vi "JHOC Data Processor.vi"(5 "Statemachine Data IN":T7={"Impulse Positions"=[], "No. Imp"=0, "Parameter Time Series"=[], "Parameter Impuls Series"=[], "Experiment Parameters"={"Freq"=0.0, "Vel"=0, "Acc"=0, "Stimulus"=""}, "Autosort File"=refnum, "Data File"={"Data Channels"=[], "Sample Rate"=0, "Channel List"=[]}, "Experiment data path"=path "/Macintosh HD/Users/patrick/Studium/Diploma Thesis/Data Analysis", "Image data path"=path "/Macintosh HD/Users/patrick/Studium/Diploma Thesis/Data Analysis", "LVS data path"=path "/Macintosh HD/Users/patrick/Studium/Diploma Thesis/Data Analysis", "Raw copy path"=path "/Macintosh HD/Users/patrick/Studium/Diploma Thesis/Data Analysis", "filename"="No file selected", "desaccading parameters"={"Tolerance"=0, "Acc Range"=0.0, "Sample Rate"=0, "Impulse Plane 2"=enum."Other", "Impulse dir"=FALSE}, "Experiment Parameters 2"={"Subject"="", "Strain"="", "Rotation plane"="", "Experimenter"="", "Trial"=0.0, "Time"=0.0}, "Excel"={"Excel._Application"=refnum, "Use Excel"=FALSE, "Worksheet SINE"=refnum, "Row SINE"=0, "Worksheet TRANS"=refnum, "Row TRANS"=0}, "Session Config File"=refnum, "Autosort Parameter Set"=1, "EMA Version"="", "desacc "={"Threshold 1 [Acc]"=1617.080808080808, "Threshold 2 [% of TH1]"=67, "tolerance"=5, "Search WD "=0.19090909090909092, " always use TH2"=TRUE, "Range"=3.2323232323232323, "Max time"=200.0, "Min time"=20.0, "Velocity Threshold"=67}, "Cycle Nr for Saccades"={"POS"=0, "NEG"=0}, "calibration name"="No file selected"} {"Parameter Time Series"."time offset" format="%.3f"; "Parameter Time Series"."Gain" format="%.1f"; "Parameter Time Series"."Offset" format="%.1f"; "Parameter Time Series"."List 1" items=["Motor-Pos", "Motor-Vel", "Lx Position-in-Head", "Ly Position-in-Head", "Lz Position-in-Head", "Lx Velocity-in-Head", "Ly Velocity-in-Head", "Lz Velocity-in-Head", "Ll Velocity-in-Head", "Lr Velocity-in-Head", "Lx Accel-in-Head", "Ly Accel-in-Head", "Lz Accel-in-Head", "Rx Position-in-Head", "Ry Position-in-Head", "Rz Position-in-Head", "Rx Velocity-in-Head", "Ry Velocity-in-Head", "Rz Velocity-in-Head", "Rl Velocity-in-Head", "Rr Velocity-in-Head", "Rx Accel-in-Head", "Ry Accel-in-Head", "Rz Accel-in-Head", "Global Trigger", "", "", ""]; "Parameter Impuls Series"."Gain" format="%.1f"; "Parameter Impuls Series"."Offset" format="%.1f"}, 8 "DC-File":path) -> (4 "Statemachine Data IN 2":T7={"Impulse Positions"=[], "No. Imp"=0, "Parameter Time Series"=[], "Parameter Impuls Series"=[], "Experiment Parameters"={"Freq"=0.0, "Vel"=0, "Acc"=0, "Stimulus"=""}, "Autosort File"=refnum, "Data File"={"Data Channels"=[], "Sample Rate"=0, "Channel List"=[]}, "Experiment data path"=path "/Macintosh HD/Users/patrick/Studium/Diploma Thesis/Data Analysis", "Image data path"=path "/Macintosh HD/Users/patrick/Studium/Diploma Thesis/Data Analysis", "LVS data path"=path "/Macintosh HD/Users/patrick/Studium/Diploma Thesis/Data Analysis", "Raw copy path"=path "/Macintosh HD/Users/patrick/Studium/Diploma Thesis/Data Analysis", "filename"="No file selected", "desaccading parameters"={"Tolerance"=0, "Acc Range"=0.0, "Sample Rate"=0, "Impulse Plane 2"=enum."Other", "Impulse dir"=FALSE}, "Experiment Parameters 2"={"Subject"="", "Strain"="", "Rotation plane"="", "Experimenter"="", "Trial"=0.0, "Time"=0.0}, "Excel"={"Excel._Application"=refnum, "Use Excel"=FALSE, "Worksheet SINE"=refnum, "Row SINE"=0, "Worksheet TRANS"=refnum, "Row TRANS"=0}, "Session Config File"=refnum, "Autosort Parameter Set"=1, "EMA Version"="", "desacc "={"Threshold 1 [Acc]"=7000.0, "Threshold 2 [% of TH1]"=60, "tolerance"=3, "Search WD "=0.1, " always use TH2"=FALSE, "Range"=2.0, "Max time"=120.0, "Min time"=20.0, "Velocity Threshold"=150}, "Cycle Nr for Saccades"={"POS"=0, "NEG"=0}, "calibration name"="No file selected"} {"Parameter Time Series"."time offset" format="%.3f"; "Parameter Time Series"."Gain" format="%.1f"; "Parameter Time Series"."Offset" format="%.1f"; "Parameter Time Series"."List 1" items=["Motor-Pos", "Motor-Vel", "Lx Position-in-Head", "Ly Position-in-Head", "Lz Position-in-Head", "Lx Velocity-in-Head", "Ly Velocity-in-Head", "Lz Velocity-in-Head", "Ll Velocity-in-Head", "Lr Velocity-in-Head", "Lx Accel-in-Head", "Ly Accel-in-Head", "Lz Accel-in-Head", "Rx Position-in-Head", "Ry Position-in-Head", "Rz Position-in-Head", "Rx Velocity-in-Head", "Ry Velocity-in-Head", "Rz Velocity-in-Head", "Rl Velocity-in-Head", "Rr Velocity-in-Head", "Rx Accel-in-Head", "Ry Accel-in-Head", "Rz Accel-in-Head", "Global Trigger", "", "", ""]; "Parameter Impuls Series"."Gain" format="%.1f"; "Parameter Impuls Series"."Offset" format="%.1f"})   [LabVIEW 2016]
uses:
  core/type-defs/TD_Statemachine-Data.ctl
  core/type-defs/TD_Time Series.ctl
  core/type-defs/TD_Impulse Parameter.ctl
  JHOC state.ctl
  core/core.lvlib
panel:
  in  "Tab Control":T1(tab)
  in  "Selected Calibration File":string
  in  "Calibration File":bool
  out "Processing":bool
  in  "3D Convention":T2(ring)=enum."Rotation Vectors"
  in  "Selected Data File":string
  in  "Data File 2":bool
  in  "Start Processing":bool
  in  "Calibration Channels":u16[][](array[ring])=[[16, 13, 10, 7, 4, 1], [15, 12, 9, 6, 3, 0], [17, 14, 11, 8, 5, 2]] items=["coil_HDX", "coil_HDY", "coil_HDZ", "coil_HTX", "coil_HTY", "coil_HTZ", "coil_LDX", "coil_LDY", "coil_LDZ", "coil_LTX", "coil_LTY", "coil_LTZ", "coil_RDX", "coil_RDY", "coil_RDZ", "coil_RTX", "coil_RTY", "coil_RTZ", "Target Hor", "Target Ver", "Target on/off", "aux input 1", "aux input 2"]
  in  "Cosines fixed":i16[][](array[numeric])
  in  "Sub Sample Once":bool
  in  "Manually enter the Field Gains":bool
  in  "Parameter Time Series":T3 {"time offset" format="%.3f"; "Gain" format="%.1f"; "Offset" format="%.1f"; "List 1" items=["Hz Position-in-Head", "Hz Velocity-in-Head", "Hy Position-in-Head", "Hy Velocity-in-Head", "Hx Position-in-Head", "Hx Velocity-in-Head", "Hl Velocity-in-Head", "Hr Velocity-in-Head", "Lx Position-in-Head", "Ly Position-in-Head", "Lz Position-in-Head", "Lx Velocity-in-Head", "Ly Velocity-in-Head", "Lz Velocity-in-Head", "Ll Velocity-in-Head", "Lr Velocity-in-Head", "Rx Position-in-Head", "Ry Position-in-Head", "Rz Position-in-Head", "Rx Velocity-in-Head", "Ry Velocity-in-Head", "Rz Velocity-in-Head", "Rl Velocity-in-Head", "Rr Velocity-in-Head", "Target on/off", "aux input 1", "aux input 2", " ", "", "", "", "Target Hor", "Target Ver", ""]}
  in  "Parameter Impuls Series":T4=[{"Color"=4652800, "Visible"=TRUE, "Channel"=1, "Invert"=FALSE, "Desaccade"=FALSE, "Offset"=0.0, "Gain"=1.0}, {"Color"=16860, "Visible"=TRUE, "Channel"=13, "Invert"=TRUE, "Desaccade"=FALSE, "Offset"=0.0, "Gain"=1.0}, {"Color"=16711680, "Visible"=TRUE, "Channel"=21, "Invert"=TRUE, "Desaccade"=FALSE, "Offset"=0.0, "Gain"=1.0}] {"Gain" format="%.1f"; "Offset" format="%.1f"; "Channel" items=["Hz Position-in-Head", "Hz Velocity-in-Head", "Hy Position-in-Head", "Hy Velocity-in-Head", "Hx Position-in-Head", "Hx Velocity-in-Head", "Hl Velocity-in-Head", "Hr Velocity-in-Head", "Lx Position-in-Head", "Ly Position-in-Head", "Lz Position-in-Head", "Lx Velocity-in-Head", "Ly Velocity-in-Head", "Lz Velocity-in-Head", "Ll Velocity-in-Head", "Lr Velocity-in-Head", "Rx Position-in-Head", "Ry Position-in-Head", "Rz Position-in-Head", "Rx Velocity-in-Head", "Ry Velocity-in-Head", "Rz Velocity-in-Head", "Rl Velocity-in-Head", "Rr Velocity-in-Head", "Target on/off", "aux input 1", "aux input 2", " ", "", "", "", "Target Hor", "Target Ver", ""]}
  in  "Export Channel List":u16[](array[ring])=[2, 11, 1, 10, 0, 9, 12, 13, 3, 4, 5, 14, 15, 16, 17, 18, 6, 7, 8, 19, 20, 21, 22, 23, 26, 27, 28, 29, 30, 31, 34, 24, 25, 38] items=["Hx Position-in-Head", "Hy Position-in-Head", "Hz Position-in-Head", "Lx Position-in-Head", "Ly Position-in-Head", "Lz Position-in-Head", "Rx Position-in-Head", "Ry Position-in-Head", "Rz Position-in-Head", "Hx Velocity-in-Head", "Hy Velocity-in-Head", "Hz Velocity-in-Head", "Hl Velocity-in-Head", "Hr Velocity-in-Head", "Lx Velocity-in-Head", "Ly Velocity-in-Head", "Lz Velocity-in-Head", "Ll Velocity-in-Head", "Lr Velocity-in-Head", "Rx Velocity-in-Head", "Ry Velocity-in-Head", "Rz Velocity-in-Head", "Rl Velocity-in-Head", "Rr Velocity-in-Head", "Target Hor", "Target Ver", "Target on/off", "aux input 1", "aux input 2", " "]
  in  "Additional channels":T5(array[cluster])=[{"offset"=0.0, "scale"=1.0, "channel select"=18}, {"offset"=0.0, "scale"=1.0, "channel select"=19}, {"offset"=0.0, "scale"=0.0060606, "channel select"=20}, {"offset"=0.0, "scale"=1.0, "channel select"=21}, {"offset"=0.0, "scale"=1.0, "channel select"=22}] {"channel select" items=["coil_HDX", "coil_HDY", "coil_HDZ", "coil_HTX", "coil_HTY", "coil_HTZ", "coil_LDX", "coil_LDY", "coil_LDZ", "coil_LTX", "coil_LTY", "coil_LTZ", "coil_RDX", "coil_RDY", "coil_RDZ", "coil_RTX", "coil_RTY", "coil_RTZ", "Target Hor", "Target Ver", "Target on/off", "aux input 1", "aux input 2"]; "scale" format="%.7f"; "offset" format="%.2f"}
  in  "Coil Channels":u16[][](array[ring])=[[0, 6, 12], [1, 7, 13], [2, 8, 14], [3, 9, 15], [4, 10, 16], [5, 11, 17]] items=["coil_HDX", "coil_HDY", "coil_HDZ", "coil_HTX", "coil_HTY", "coil_HTZ", "coil_LDX", "coil_LDY", "coil_LDZ", "coil_LTX", "coil_LTY", "coil_LTZ", "coil_RDX", "coil_RDY", "coil_RDZ", "coil_RTX", "coil_RTY", "coil_RTZ", "Target Hor", "Target Ver", "Target on/off", "aux input 1", "aux input 2"]
  in  "DAQ data setup":T6={"Input Channels"=[{"channel name"="coil_HDX", "channel number"=0.0}, {"channel name"="coil_HDY", "channel number"=1.0}, {"channel name"="coil_HDZ", "channel number"=2.0}, {"channel name"="coil_HTX", "channel number"=3.0}, {"channel name"="coil_HTY", "channel number"=4.0}, {"channel name"="coil_HTZ", "channel number"=5.0}, {"channel name"="coilLDX", "channel number"=6.0}, {"channel name"="coil_LDY", "channel number"=7.0}, {"channel name"="coil_LDZ", "channel number"=8.0}, {"channel name"="coil_LTX", "channel number"=9.0}, {"channel name"="coil_LTY", "channel number"=10.0}, {"channel name"="coil_LTZ", "channel number"=11.0}, {"channel name"="coil_RDX", "channel number"=12.0}, {"channel name"="coil_RDY", "channel number"=13.0}, {"channel name"="coil_RDZ", "channel number"=14.0}, {"channel name"="coil_RTX", "channel number"=15.0}, {"channel name"="coil_RTY", "channel number"=16.0}, {"channel name"="coil_RTZ", "channel number"=17.0}], "Sample Rate"=1000.0}
  in  "plot length":i32=15000
  in  "Channel \nplot":u16[](array[ring])=[7, 8, 10, 11, 1, 2] items=["coil_HDX", "coil_HDY", "coil_HDZ", "coil_HTX", "coil_HTY", "coil_HTZ", "coil_LDX", "coil_LDY", "coil_LDZ", "coil_LTX", "coil_LTY", "coil_LTZ", "coil_RDX", "coil_RDY", "coil_RDZ", "coil_RTX", "coil_RTY", "coil_RTZ", "Target Hor", "Target Ver", "Target on/off", "aux input 1", "aux input 2"]
  out "DAQ calibration setup":T6={"Input Channels"=[{"channel name"="chairpos", "channel number"=1.0}, {"channel name"="coil_RDY", "channel number"=2.0}, {"channel name"="coil_RDZ", "channel number"=3.0}, {"channel name"="coil_RDX", "channel number"=4.0}, {"channel name"="coil_RTY", "channel number"=5.0}, {"channel name"="coil_RTZ", "channel number"=6.0}, {"channel name"="coil_RTX", "channel number"=7.0}, {"channel name"="coil_HDY", "channel number"=8.0}, {"channel name"="coil_HDZ", "channel number"=9.0}, {"channel name"="coil_HDX", "channel number"=10.0}, {"channel name"="coil_LDY", "channel number"=11.0}, {"channel name"="coil_LDZ", "channel number"=12.0}, {"channel name"="coil_LDX", "channel number"=13.0}, {"channel name"="coil_LTY", "channel number"=14.0}, {"channel name"="coil_LTZ", "channel number"=15.0}, {"channel name"="coil_LTX", "channel number"=16.0}, {"channel name"="coil_HTY", "channel number"=17.0}, {"channel name"="coil_HTZ", "channel number"=18.0}, {"channel name"="coil_HTX", "channel number"=19.0}, {"channel name"="chairvel", "channel number"=20.0}, {"channel name"="button", "channel number"=22.0}, {"channel name"="accel_head", "channel number"=25.0}, {"channel name"="ascension_x", "channel number"=33.0}, {"channel name"="ascension_y", "channel number"=34.0}, {"channel name"="ascension_z", "channel number"=35.0}, {"channel name"="ascension_q0", "channel number"=36.0}, {"channel name"="ascension_q1", "channel number"=37.0}, {"channel name"="ascension_q2", "channel number"=38.0}, {"channel name"="ascension_q3", "channel number"=39.0}, {"channel name"="led_code", "channel number"=40.0}], "Sample Rate"=1000.0}
  in  "Data File":T8 {"Data -> Plot" format="%.2f"; "Data -> Additional" format="%.2f"; "Data -> 3D Coil" format="%.2f"}
  in  "All Data":T9={"Data Channels"=[], "Sample Rate"=0, "Channel List"=["Hx Position-in-Head", "Hy Position-in-Head", "Hz Position-in-Head", "Lx Position-in-Head", "Ly Position-in-Head", "Lz Position-in-Head", "Rx Position-in-Head", "Ry Position-in-Head", "Rz Position-in-Head", "Hx Velocity-in-Head", "Hy Velocity-in-Head", "Hz Velocity-in-Head", "Hl Velocity-in-Head", "Hr Velocity-in-Head", "Lx Velocity-in-Head", "Ly Velocity-in-Head", "Lz Velocity-in-Head", "Ll Velocity-in-Head", "Lr Velocity-in-Head", "Rx Velocity-in-Head", "Ry Velocity-in-Head", "Rz Velocity-in-Head", "Rl Velocity-in-Head", "Rr Velocity-in-Head", "coil_HTX", "chairvel", "button", " "]} {"Data Channels" format="%.2f"}
  # "NOTE: EMPTY STRING ALWAYS AT END"
  # "JHOC Data Processor"
  # "By Americo A. Migliaccio\nand Patrick P. Huebner \nMarch 2014 ver 2.0"
  # "Head coil                             Left eye coil                        Right eye coil"
  # "DX\n\nDY\n\nDZ\n\nTX\n\nTY\n\nTZ"
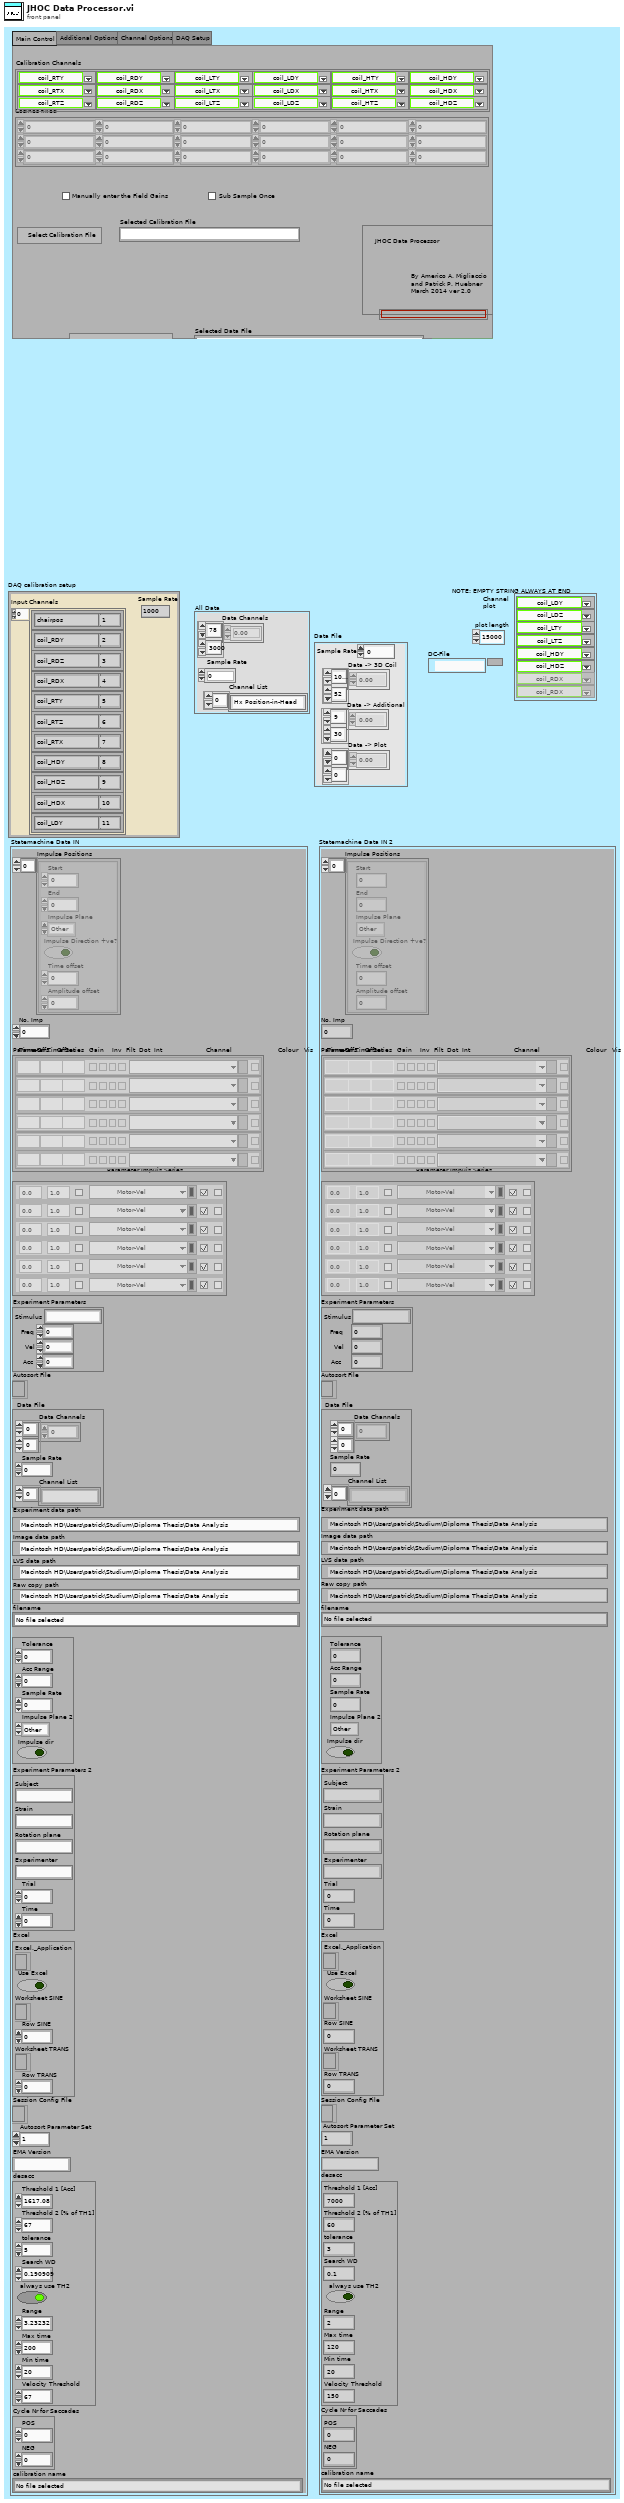
[diagram p1: front panel]
types:
  T1 = enum32{"Main Control", "Additional Options", "Channel Options", "DAQ Setup"}
  T2 = enum16{"Rotation Matrix", "Rotation Vectors", "Quaternions", "Fick Angles", "Helmholtz Angles"}
  T3 = typedef "core.lvlib/TD_Time Series.ctl" = cluster{"time offset":dbl, "Offset":dbl, "Gain":dbl, "inverse":bool, "filter data":bool, "dots":bool, "interpolate":bool, "List 1":u16, "Color Box":u32, "Boolean":bool}[]
  T4 = typedef "core.lvlib/TD_Impulse Parameter.ctl" = cluster{"Color":u32, "Visible":bool, "Channel":u16, "Invert":bool, "Desaccade":bool, "Offset":dbl, "Gain":dbl}[]
  T5 = cluster{"offset":dbl, "scale":dbl, "channel select":u16}[]
  T6 = cluster{"Input Channels":cluster{"channel name":string, "channel number":dbl}[], "Sample Rate":dbl}
  T7 = typedef "core.lvlib/TD_Statemachine-Data.ctl" = cluster{"Impulse Positions":cluster{"Start":i32, "End":i32, "Impulse Plane":enum16{"Other", "Yaw", "Pitch", "Roll", "LARP", "RALP"}, "Impulse Direction +ve?":bool, "Time offset":i32, "Amplitude offset":dbl}[], "No. Imp":i32, "Parameter Time Series":T3, "Parameter Impuls Series":T4, "Experiment Parameters":cluster{"Freq":dbl, "Vel":i32, "Acc":i32, "Stimulus":string}, "Autosort File":refnum<file>, "Data File":cluster{"Data Channels":dbl[][], "Sample Rate":i32, "Channel List":string[]}, "Experiment data path":path, "Image data path":path, "LVS data path":path, "Raw copy path":path, "filename":string, "desaccading parameters":cluster{"Tolerance":i32, "Acc Range":dbl, "Sample Rate":i32, "Impulse Plane 2":enum16{"Other", "Yaw", "Pitch", "Roll", "LARP", "RALP"}, "Impulse dir":bool}, "Experiment Parameters 2":cluster{"Subject":string, "Strain":string, "Rotation plane":string, "Experimenter":string, "Trial":dbl, "Time":dbl}, "Excel":cluster{"Excel._Application":refnum<k7>, "Use Excel":bool, "Worksheet SINE":refnum<k7>, "Row SINE":i32, "Worksheet TRANS":refnum<k7>, "Row TRANS":i32}, "Session Config File":refnum<file>, "Autosort Parameter Set":i32, "EMA Version":string, "desacc ":cluster{"Threshold 1 [Acc]":dbl, "Threshold 2 [% of TH1]":i32, "tolerance":i32, "Search WD ":dbl, " always use TH2":bool, "Range":dbl, "Max time":dbl, "Min time":dbl, "Velocity Threshold":i32}, "Cycle Nr for Saccades":cluster{"POS":i32, "NEG":i32}, "calibration name":string}
  T8 = cluster{"Sample Rate":i32, "Data -> 3D Coil":dbl[][], "Data -> Additional":dbl[][], "Data -> Plot":dbl[][]}
  T9 = cluster{"Data Channels":dbl[][], "Sample Rate":i32, "Channel List":string[]}
  T10 = typedef "JHOC state.ctl" = enum16{"Panel Monitoring", "Calculate 6 Field/Int Rot Matrix", "SubSample", "Initialize", "Read 6 Field/Int Calibration File", "Read 6 Field/Int Data File", "Sort 6 Field/Int Channels", "Export Channels", "Stop", "Quit"}
  T11 = enum16{"Position in Space", "Position in Head", "Position in Eye", "Velocity in Space", "Velocity in Head", "Velocity in Eye", "Acceleration in Space", "Acceleration in Head"}
  T12 = cluster{"Freq":dbl, "Vel":i32, "Acc":i32, "Stimulus":string}
  T13 = cluster{"DAQ data setup":cluster{"Input Channels":cluster{"channel name":string, "channel number":dbl}[], "Sample Rate":dbl}, "Coil Channels":u16[][], "Additional channels":cluster{"offset":dbl, "scale":dbl, "channel select":u16}[], "Selected Calibration File":string, "Selected Data File":string, "Cosines fixed":i16[][], "Data File":cluster{"Sample Rate":i32, "Data -> 3D Coil":dbl[][], "Data -> Additional":dbl[][], "Data -> Plot":dbl[][]}, "All Data":cluster{"Data Channels":dbl[][], "Sample Rate":i32, "Channel List":string[]}, "Channel \nplot":u16[], "Calibration Channels":u16[][], "Auto load calibration file":path}
  T14 = cluster{"DAQ calibration setup":cluster{"Input Channels":cluster{"channel name":string, "channel number":dbl}[], "Sample Rate":dbl}, "Calibration Channels":u16[][]}
  T15 = cluster{"channel name":string, "channel number":dbl}[]
  T16 = cluster{"channel name":string, "channel number":dbl}
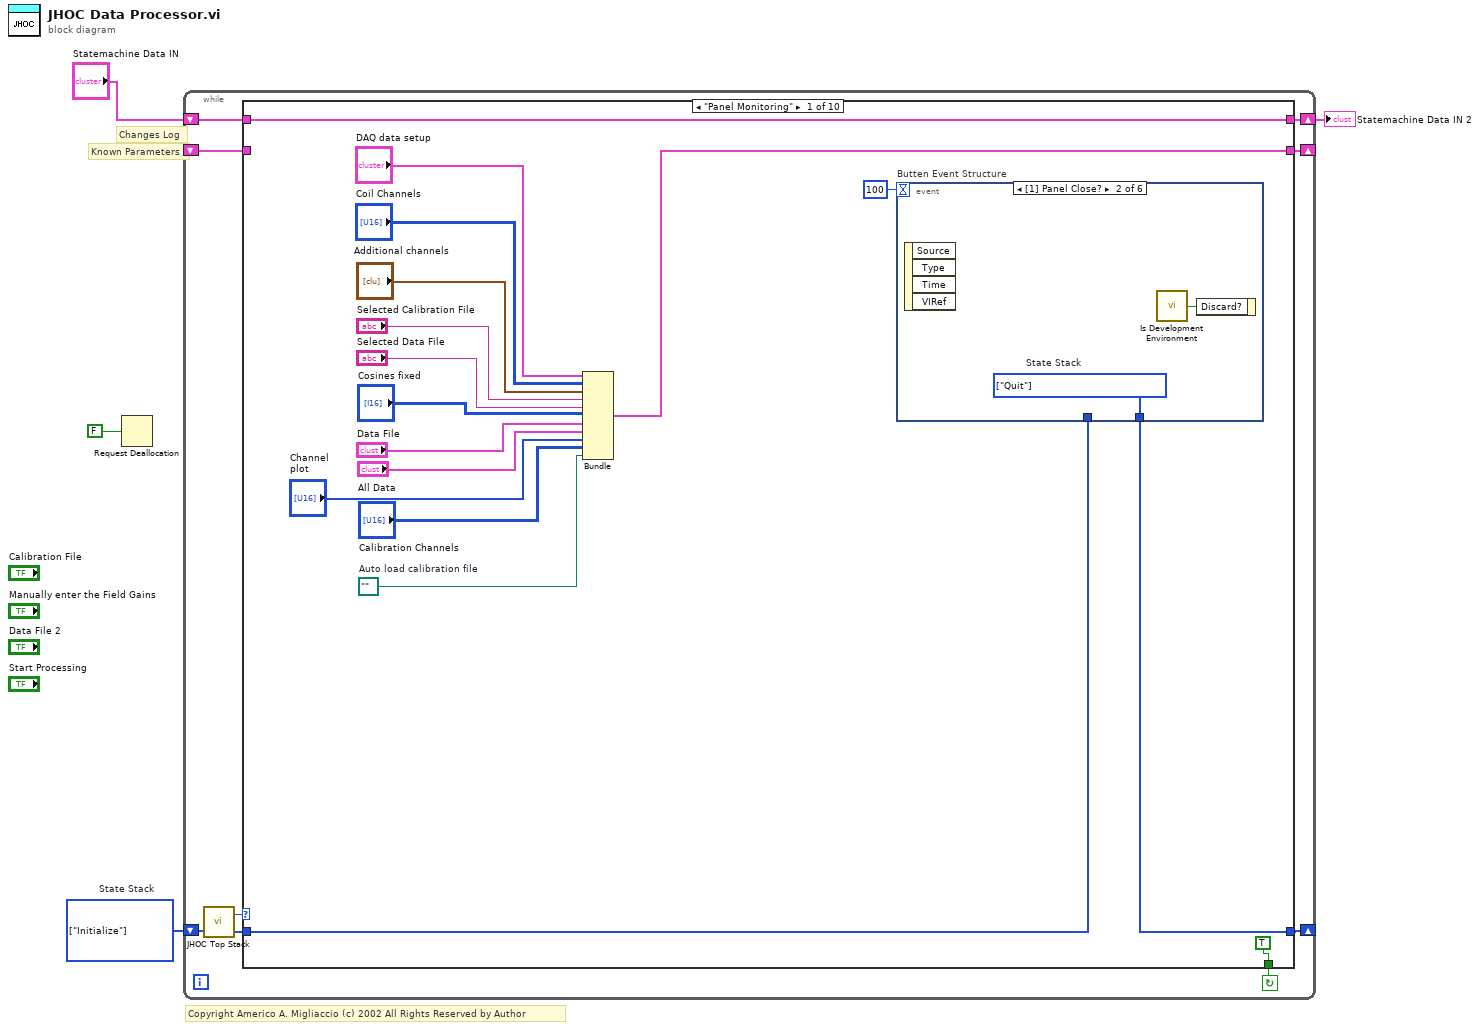
[diagram p0: block diagram]
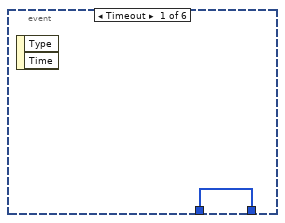
[diagram p2: hidden frame]
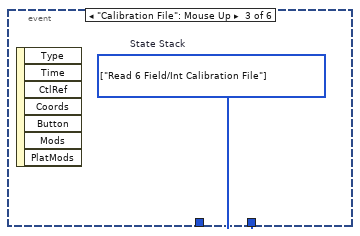
[diagram p3: hidden frame]
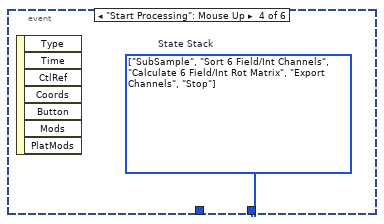
[diagram p4: hidden frame]
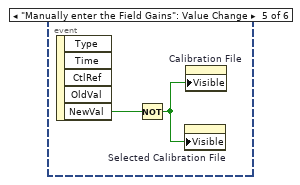
[diagram p5: hidden frame]
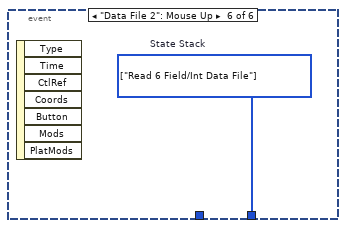
[diagram p6: hidden frame]
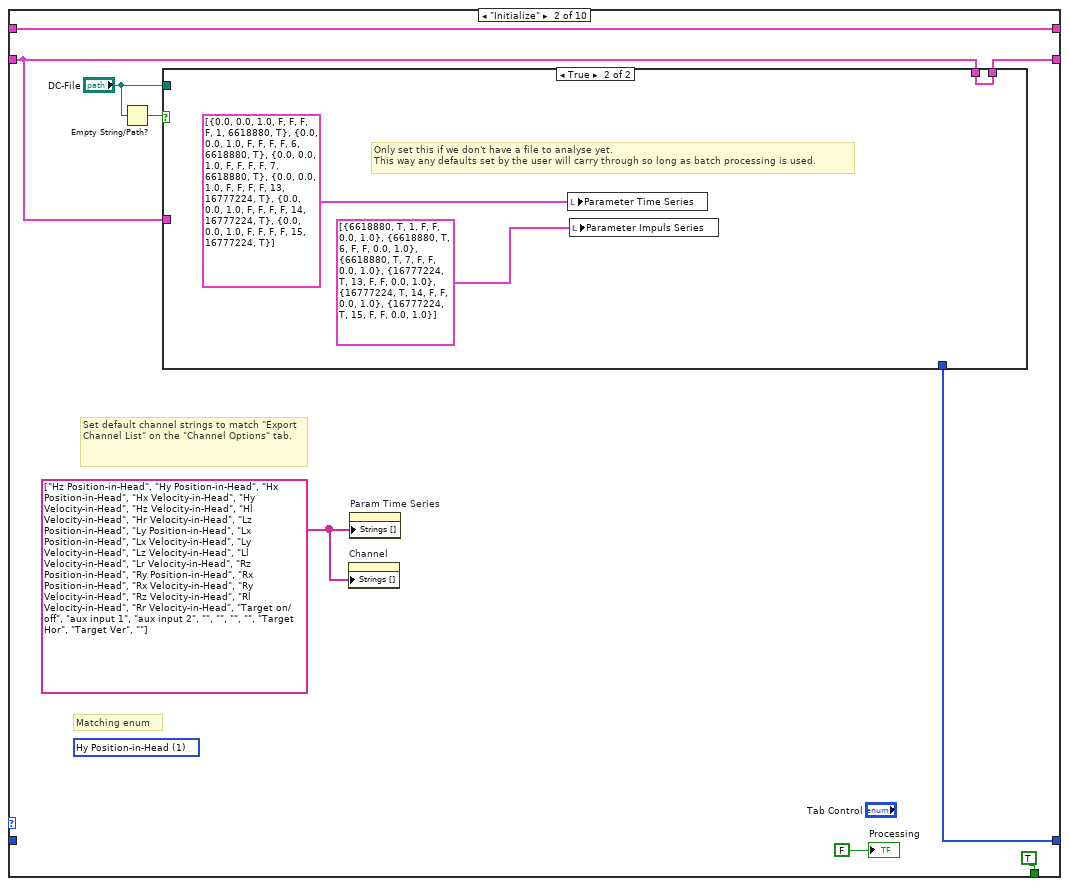
[diagram p7: hidden frame]
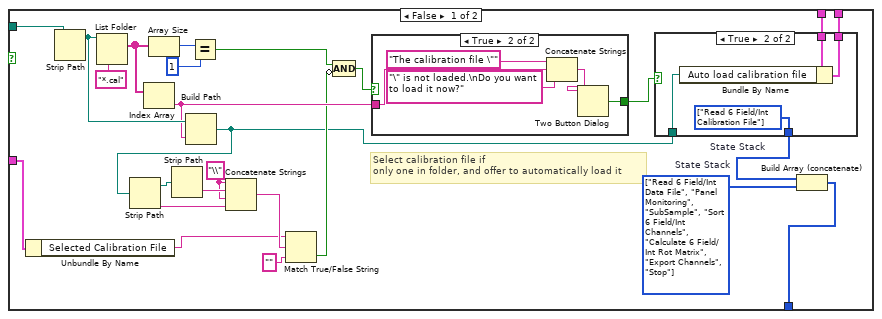
[diagram p8: hidden frame]
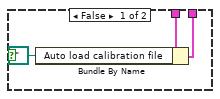
[diagram p9: hidden frame]
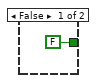
[diagram p10: hidden frame]
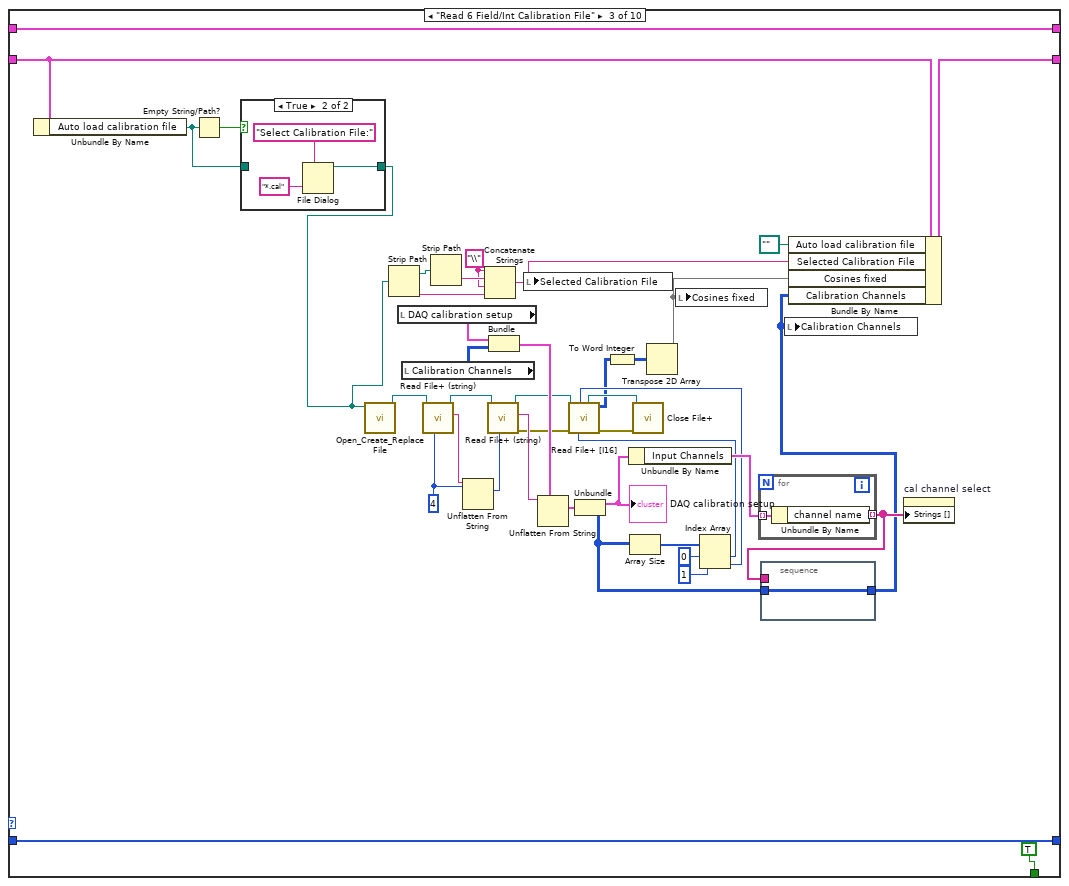
[diagram p11: hidden frame]
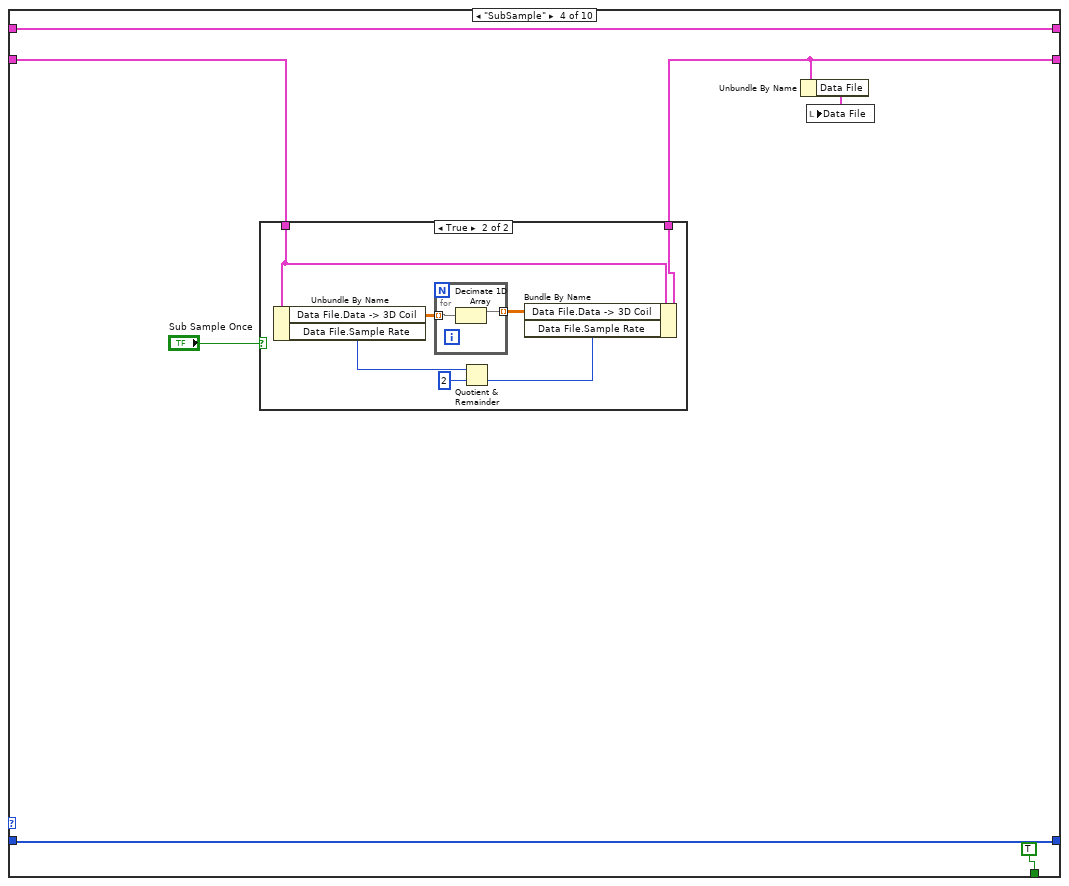
[diagram p13: hidden frame]
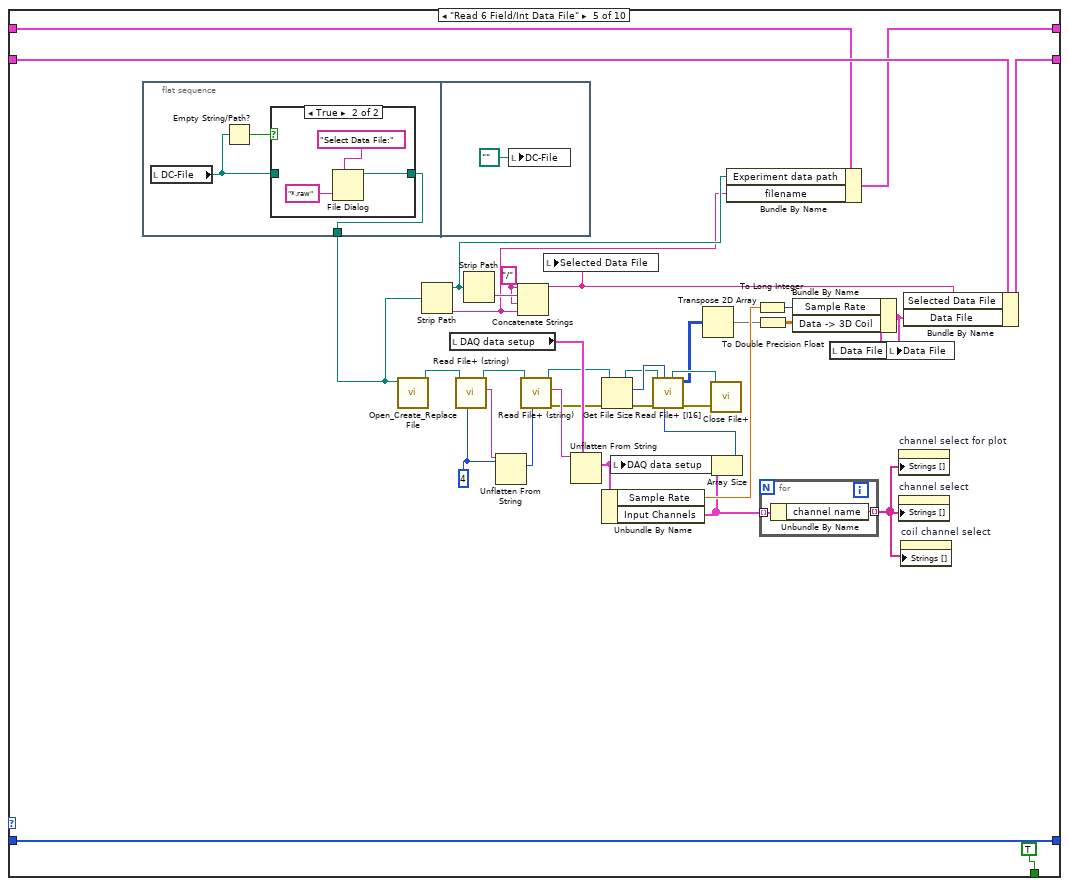
[diagram p15: hidden frame]
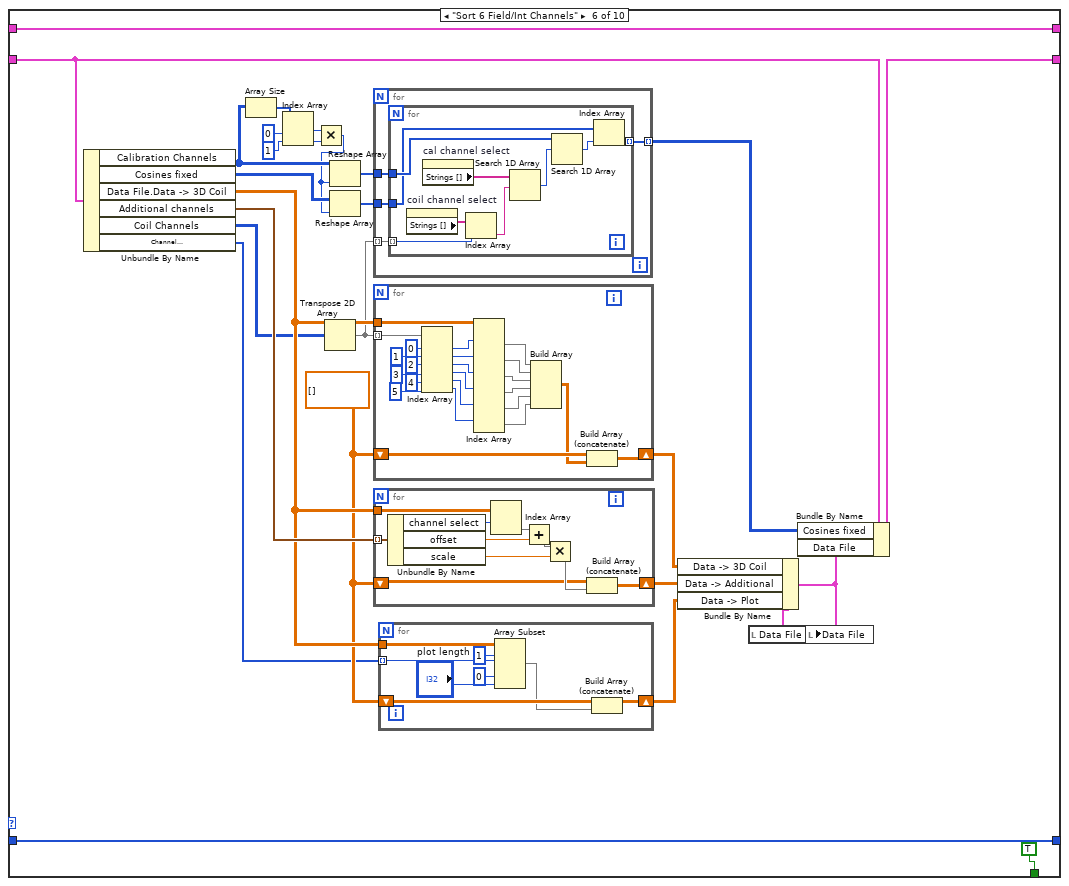
[diagram p17: hidden frame]
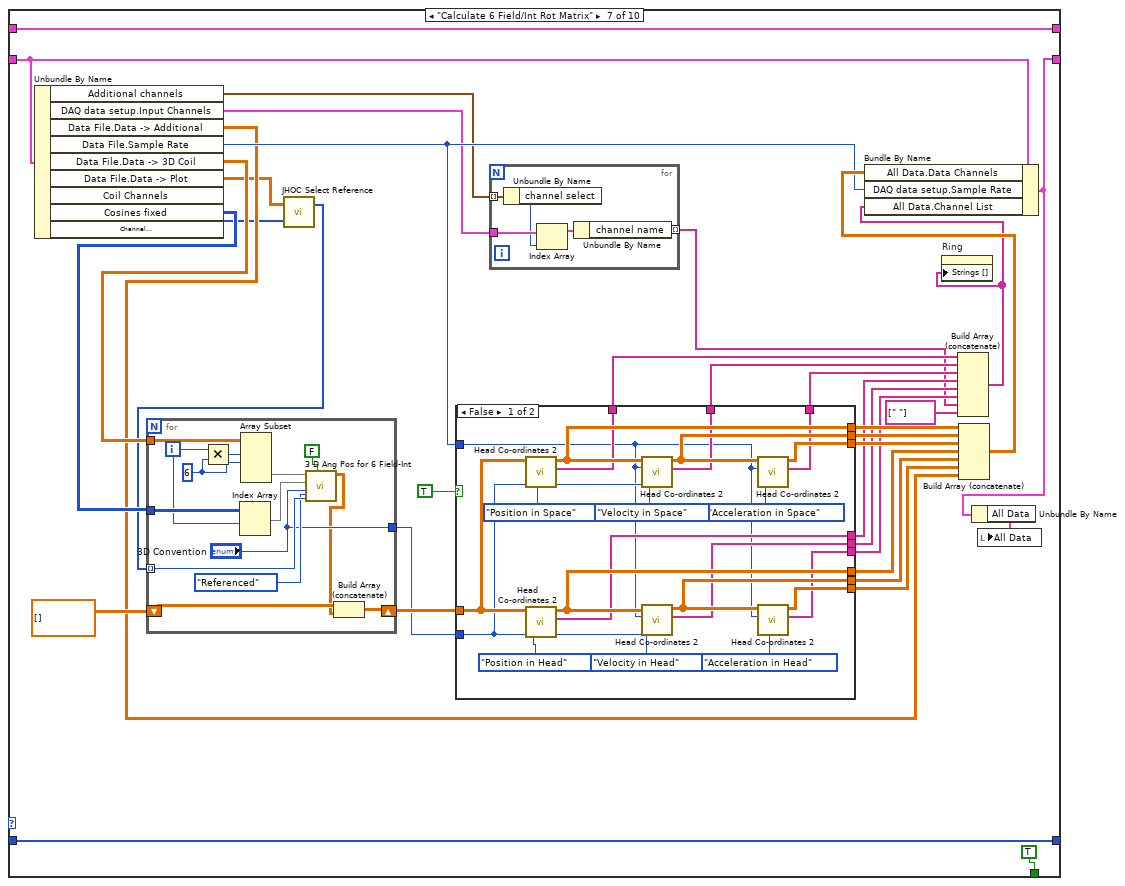
[diagram p18: hidden frame]
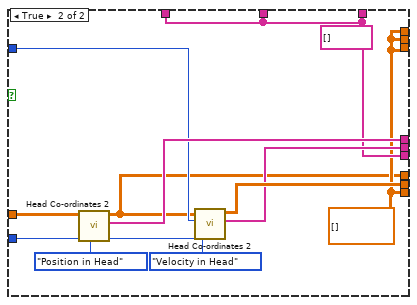
[diagram p19: hidden frame]
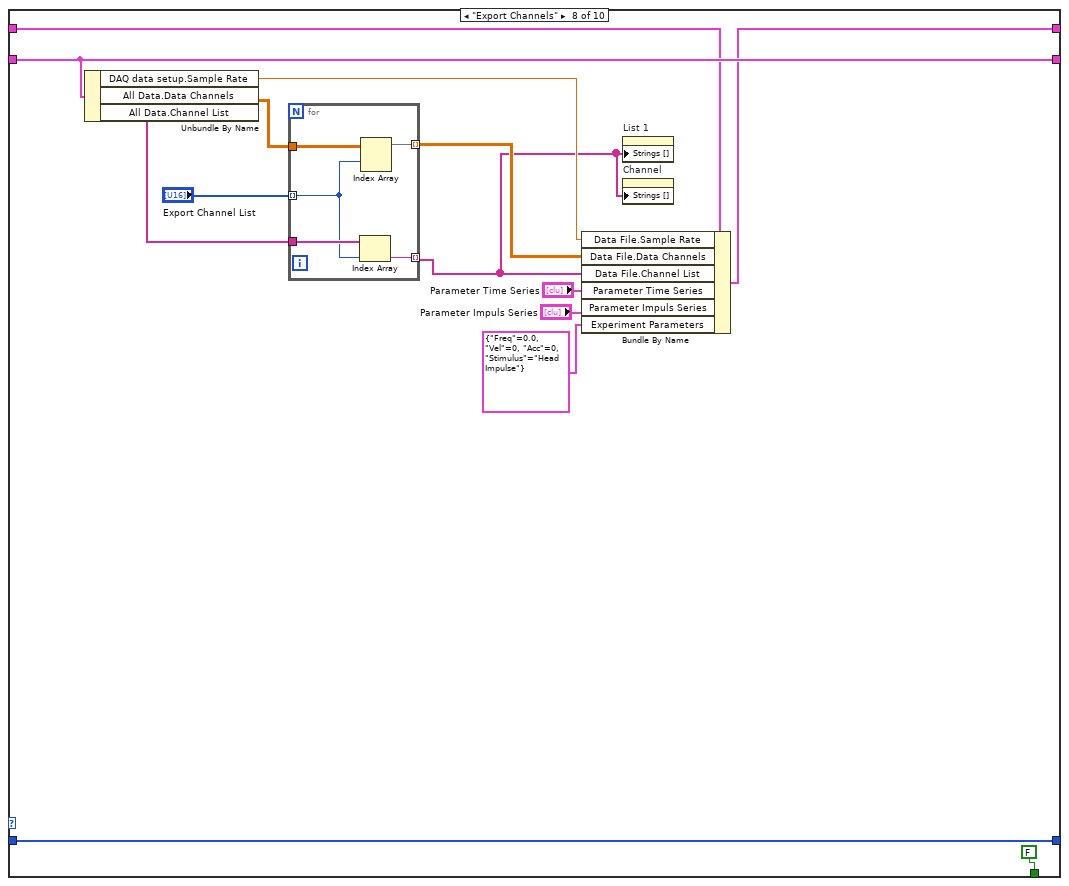
[diagram p20: hidden frame]
diagram:
  w4 = T10[] [enum."Initialize"] items=["Panel Monitoring", "Calculate 6 Field/Int Rot Matrix", "SubSample", "Initialize", "Read 6 Field/Int Calibration File", "Read 6 Field/Int Data File", "Sort 6 Field/Int Channels", "Export Channels", "Stop", "Quit"]  # State Stack
  # "Copyright Americo A. Migliaccio (c) 2002 All Rights Reserved by Author"
  # "Known Parameters"
  # "Changes Log"
  n1 = Request Deallocation(FALSE ("flag")) -> ()
  n2 = while {
    shift-left: _ -> [w9]
    shift-right: [w8] -> _
    shift-left: w4 -> [w13]
    shift-right: [w11] -> _
    shift-right: [w5] -> w1
    shift-left: "Statemachine Data IN" -> [w6]
    stop <- w10 continue-if-true
    n3 = call "JHOC Top Stack.vi"("State Stack (in)"=w13) -> ("State Stack (out)"=w12:T10[], "State 4"=w7:T10)  [unwired: 1 in]
    n4 = case shown="\"Panel Monitoring\"" w7 {
      tunnel: w12 -> [w14 _ w89 w138 w154 w225 w316 w381 w390 w394]
      tunnel: [w17 w41 w89 w138 w154 w225 w316 w381 w390 w394] -> w11
      tunnel: [TRUE TRUE TRUE TRUE TRUE TRUE TRUE FALSE FALSE FALSE] -> w10
      tunnel: [w27 w42 w128 w140 w189 w224 w302 w378 w388 w392] -> w8
      tunnel: w9 -> [_ w40 w94 w142 w188 w226 w312 w378 w388 w392]
      tunnel: w6 -> [w18 w45 w95 w137 w156 w201 w282 w373 w387 w391]
      tunnel: [w18 w45 w95 w137 w155 w201 w282 w372 w387 w391] -> w5
      frame "Panel Monitoring" {
        w15 = path ""  # Auto load calibration file
        n5 = Bundle("DAQ data setup"="DAQ data setup", "Coil Channels"="Coil Channels", "Additional channels"="Additional channels", "Selected Calibration File"="Selected Calibration File", "Selected Data File"="Selected Data File", "Cosines fixed"="Cosines fixed", "Data File"="Data File", "All Data"="All Data", "Channel \nplot"="Channel \nplot", "Calibration Channels"="Calibration Channels", "Auto load calibration file"=w15) -> (w27:T13)  [unwired: 1 in]
        n6 = event "Butten Event Structure" shown="[1] Panel Close?" {
          selector: _ -> [_ _ _ _ _ _]
          dyn-events: _ -> [_ _ _ _ _ _]
          timeout: 100 -> [_ _ _ _ _ _]
          tunnel: [w31 w33 w34 w35 _ w38] -> w17
          tunnel: w14 -> [w31 _ _ _ _ _]
          event Timeout {
            n7 = event-data() -> ()  [unwired: 1 in, 2 out]
          }
          event Panel Close? {
            w33 = T10[] [enum."Quit"] items=["Panel Monitoring", "Calculate 6 Field/Int Rot Matrix", "SubSample", "Initialize", "Read 6 Field/Int Calibration File", "Read 6 Field/Int Data File", "Sort 6 Field/Int Channels", "Export Channels", "Stop", "Quit"]  # State Stack
            n8 = event-data() -> ()  [unwired: 1 in, 4 out]
            n9 = call <userlib>:"Is Development Environment.vi"() -> ("exe?"=w32:bool)  [unwired: 5 in]
            n10 = event-data("Discard?"=w32) -> ()  [unwired: 1 in, 1 out]
          }
          event "Calibration File": Mouse Up {
            w34 = T10[] [enum."Read 6 Field/Int Calibration File"] items=["Panel Monitoring", "Calculate 6 Field/Int Rot Matrix", "SubSample", "Initialize", "Read 6 Field/Int Calibration File", "Read 6 Field/Int Data File", "Sort 6 Field/Int Channels", "Export Channels", "Stop", "Quit"]  # State Stack
            n11 = event-data() -> ()  [unwired: 1 in, 7 out]
          }
          event "Start Processing": Mouse Up {
            w35 = T10[] [enum."SubSample", enum."Sort 6 Field/Int Channels", enum."Calculate 6 Field/Int Rot Matrix", enum."Export Channels", enum."Stop"] items=["Panel Monitoring", "Calculate 6 Field/Int Rot Matrix", "SubSample", "Initialize", "Read 6 Field/Int Calibration File", "Read 6 Field/Int Data File", "Sort 6 Field/Int Channels", "Export Channels", "Stop", "Quit"]  # State Stack
            n12 = event-data() -> ()  [unwired: 1 in, 7 out]
          }
          event "Manually enter the Field Gains": Value Change {
            n13 = event-data() -> ("NewVal"=w36:bool)  [unwired: 1 in, 4 out]
            n14 = Not(x=w36) -> (.not. x?=w37:bool)
            n15 = property on="Selected Calibration File" class="Str"("Visible"=w37) -> ()  [unwired: 2 in, 2 out]
            n16 = property on="Calibration File" class="Bool (strict)"("Visible"=w37) -> ()  [unwired: 2 in, 2 out]
          }
          event "Data File 2": Mouse Up {
            w38 = T10[] [enum."Read 6 Field/Int Data File"] items=["Panel Monitoring", "Calculate 6 Field/Int Rot Matrix", "SubSample", "Initialize", "Read 6 Field/Int Calibration File", "Read 6 Field/Int Data File", "Sort 6 Field/Int Channels", "Export Channels", "Stop", "Quit"]  # State Stack
            n17 = event-data() -> ()  [unwired: 1 in, 7 out]
          }
        }
      }
      frame "Initialize" {
        (unwired) u16 1 items=["Hz Position-in-Head", "Hy Position-in-Head", "Hx Position-in-Head", "Hx Velocity-in-Head", "Hy Velocity-in-Head", "Hz Velocity-in-Head", "Hl Velocity-in-Head", "Hr Velocity-in-Head", "Lx Position-in-Head", "Ly Position-in-Head", "Lz Position-in-Head", "Lx Velocity-in-Head", "Ly Velocity-in-Head", "Lz Velocity-in-Head", "Ll Velocity-in-Head", "Lr Velocity-in-Head", "Rz Position-in-Head", "Ry Position-in-Head", "Rx Position-in-Head", "Rx Velocity-in-Head", "Ry Velocity-in-Head", "Rz Velocity-in-Head", "Rl Velocity-in-Head", "Rr Velocity-in-Head", "Target on/off", "aux input 1", "aux input 2", "", "", "", "", "Target Hor", "Target Ver", ""] ("Channel")
        w39 = string[] ["Hz Position-in-Head", "Hy Position-in-Head", "Hx Position-in-Head", "Hx Velocity-in-Head", "Hy Velocity-in-Head", "Hz Velocity-in-Head", "Hl Velocity-in-Head", "Hr Velocity-in-Head", "Lz Position-in-Head", "Ly Position-in-Head", "Lx Position-in-Head", "Lx Velocity-in-Head", "Ly Velocity-in-Head", "Lz Velocity-in-Head", "Ll Velocity-in-Head", "Lr Velocity-in-Head", "Rz Position-in-Head", "Ry Position-in-Head", "Rx Position-in-Head", "Rx Velocity-in-Head", "Ry Velocity-in-Head", "Rz Velocity-in-Head", "Rl Velocity-in-Head", "Rr Velocity-in-Head", "Target on/off", "aux input 1", "aux input 2", "", "", "", "", "Target Hor", "Target Ver", ""]
        # "Matching enum"
        # "Set default channel strings to match \"Export Channel List\" on the \"Channel Options\" tab."
        n18 = Empty String/Path?(string/path="DC-File") -> (empty?=w43:bool)
        n19 = case shown="True" w43 {
          tunnel: w40 -> [w68 _]
          tunnel: "DC-File" -> [w67 _]
          tunnel: w40 -> [w64 w88]
          tunnel: [w62 w88] -> w42
          tunnel: [w48 _] -> w41
          frame False {
            w49 = T10[] [enum."Read 6 Field/Int Data File", enum."Panel Monitoring", enum."SubSample", enum."Sort 6 Field/Int Channels", enum."Calculate 6 Field/Int Rot Matrix", enum."Export Channels", enum."Stop"] items=["Panel Monitoring", "Calculate 6 Field/Int Rot Matrix", "SubSample", "Initialize", "Read 6 Field/Int Calibration File", "Read 6 Field/Int Data File", "Sort 6 Field/Int Channels", "Export Channels", "Stop", "Quit"]  # State Stack
            w55 = "\\" ("Substring")
            # "Select calibration file if\nonly one in folder, and offer to automatically load it"
            n20 = Unbundle By Name(w68) -> ("Selected Calibration File"=w51:string)
            n21 = Strip Path(path=w67) -> (stripped path=w69:path)  [unwired: 1 out]
            n22 = List Folder(path=w69, pattern="*.cal") -> (filenames=w70:string[])  [unwired: 2 in, 3 out]
            n23 = Index Array(array=w70) -> (element=w66:string)  [unwired: 1 in]
            n24 = Array Size(array=w70) -> (size(s)=w72:i32)
            n25 = Build Path(base path=w69, name or relative path=w66) -> (appended path=w53:path)
            n26 = Strip Path(path=w53) -> (stripped path=w57:path, name=w54:string)
            n27 = Strip Path(path=w57) -> (name=w56:string)  [unwired: 1 out]
            n28 = Equal?(x=w72, y=1) -> (x = y?=w61:bool)
            n29 = Concatenate Strings(w55, w56, w55, w54) -> (w52:string)
            n30 = Match True/False String(2:"" ("false string"), 3:w52, 4:w51) -> (0:w59:bool)  [unwired: 1 out]
            n31 = Compound Arithmetic op=AND(w61, invert w59) -> (w60:bool)
            n32 = case shown="True" w60 {
              tunnel: w66 -> [_ w84]
              tunnel: [FALSE ("T button?") w81] -> w63
              frame False {
              }
              frame True {
                n33 = Concatenate Strings("The calibration file \"" ("string"), w84, "\" is not loaded.\nDo you want to load it now?" ("string")) -> (w82:string)
                n34 = Two Button Dialog(message=w82) -> (T button?=w81:bool)  [unwired: 2 in]
              }
            }
            n35 = case shown="True" w63 {
              tunnel: w64 -> [w75 w79]
              tunnel: [w74 w78] -> w62
              tunnel: w53 -> [_ w77]
              tunnel: [_ w76] -> w50
              frame False {
                n36 = Bundle By Name(cluster=w75, "Auto load calibration file"=path "") -> (w74:T13)
              }
              frame True {
                w76 = T10[] [enum."Read 6 Field/Int Calibration File"] items=["Panel Monitoring", "Calculate 6 Field/Int Rot Matrix", "SubSample", "Initialize", "Read 6 Field/Int Calibration File", "Read 6 Field/Int Data File", "Sort 6 Field/Int Channels", "Export Channels", "Stop", "Quit"]  # State Stack
                n37 = Bundle By Name(cluster=w79, "Auto load calibration file"=w77) -> (w78:T13)
              }
            }
            n38 = Build Array (concatenate)(w50, w49) -> (w48:T10[])
          }
          frame True {
            # "Only set this if we don't have a file to analyse yet.\nThis way any defaults set by the user will carry through so long as batch processing is used."
            n39 = local write "Parameter Time Series"(T3 [{"time offset"=0.0, "Offset"=0.0, "Gain"=1.0, "inverse"=FALSE, "filter data"=FALSE, "dots"=FALSE, "interpolate"=FALSE, "List 1"=1, "Color Box"=6618880, "Boolean"=TRUE}, {"time offset"=0.0, "Offset"=0.0, "Gain"=1.0, "inverse"=FALSE, "filter data"=FALSE, "dots"=FALSE, "interpolate"=FALSE, "List 1"=6, "Color Box"=6618880, "Boolean"=TRUE}, {"time offset"=0.0, "Offset"=0.0, "Gain"=1.0, "inverse"=FALSE, "filter data"=FALSE, "dots"=FALSE, "interpolate"=FALSE, "List 1"=7, "Color Box"=6618880, "Boolean"=TRUE}, {"time offset"=0.0, "Offset"=0.0, "Gain"=1.0, "inverse"=FALSE, "filter data"=FALSE, "dots"=FALSE, "interpolate"=FALSE, "List 1"=13, "Color Box"=16777224, "Boolean"=TRUE}, {"time offset"=0.0, "Offset"=0.0, "Gain"=1.0, "inverse"=FALSE, "filter data"=FALSE, "dots"=FALSE, "interpolate"=FALSE, "List 1"=14, "Color Box"=16777224, "Boolean"=TRUE}, {"time offset"=0.0, "Offset"=0.0, "Gain"=1.0, "inverse"=FALSE, "filter data"=FALSE, "dots"=FALSE, "interpolate"=FALSE, "List 1"=15, "Color Box"=16777224, "Boolean"=TRUE}] ("Parameter Time Series")) -> ()
            n40 = local write "Parameter Impuls Series"(T4 [{"Color"=6618880, "Visible"=TRUE, "Channel"=1, "Invert"=FALSE, "Desaccade"=FALSE, "Offset"=0.0, "Gain"=1.0}, {"Color"=6618880, "Visible"=TRUE, "Channel"=6, "Invert"=FALSE, "Desaccade"=FALSE, "Offset"=0.0, "Gain"=1.0}, {"Color"=6618880, "Visible"=TRUE, "Channel"=7, "Invert"=FALSE, "Desaccade"=FALSE, "Offset"=0.0, "Gain"=1.0}, {"Color"=16777224, "Visible"=TRUE, "Channel"=13, "Invert"=FALSE, "Desaccade"=FALSE, "Offset"=0.0, "Gain"=1.0}, {"Color"=16777224, "Visible"=TRUE, "Channel"=14, "Invert"=FALSE, "Desaccade"=FALSE, "Offset"=0.0, "Gain"=1.0}, {"Color"=16777224, "Visible"=TRUE, "Channel"=15, "Invert"=FALSE, "Desaccade"=FALSE, "Offset"=0.0, "Gain"=1.0}] ("Parameter Impuls Series")) -> ()
          }
        }
        n41 = property on="Channel" class="Ring (strict)"("Strings []"=w39) -> ()  [unwired: 2 in, 2 out]
        n42 = property on="Param Time Series" class="Ring (strict)"("Strings []"=w39) -> ()  [unwired: 2 in, 2 out]
        "Processing" <- FALSE ("Processing")
      }
      frame "Read 6 Field/Int Calibration File" {
        w118 = 4 ("count")
        w125 = "\\" ("Substring")
        n43 = Unbundle By Name(w94) -> ("Auto load calibration file"=w92:path)
        n44 = Empty String/Path?(string/path=w92) -> (empty?=w93:bool)
        n45 = case shown="True" w93 {
          tunnel: w92 -> [w130 _]
          tunnel: [w130 w131] -> w91
          frame False {
          }
          frame True {
            n46 = File Dialog(6:"*.cal" ("pattern"), 7:"Select Calibration File:" ("prompt")) -> (3:w131:path)  [unwired: 5 in, 3 out]
          }
        }
        n47 = call <vilib>:"Open_Create_Replace File.vi"("file path"=w91) -> ("refnum"=w121:refnum<file>)  [unwired: 7 in, 3 out]
        n48 = Strip Path(path=w91) -> (stripped path=w127:path, name=w124:string)
        n49 = local read "DAQ calibration setup"() -> (w113:T6)
        n50 = local read "Calibration Channels"() -> (w114:u16[][])
        n51 = call <vilib>:"Read File+ (string).vi"("count"=w118, "refnum"=w121) -> ("string"=w119:string, "dup refnum"=w120:refnum<file>)  [unwired: 5 in, 3 out]
        n52 = Strip Path(path=w127) -> (name=w126:string)  [unwired: 1 out]
        n53 = Unflatten From String(type=w118, binary string=w119) -> (value=w117:i32)  [unwired: 3 in, 2 out]
        n54 = Concatenate Strings(w125, w126, w125, w124) -> (w123:string)
        n55 = call <vilib>:"Read File+ (string).vi"("count"=w117, "refnum"=w120) -> ("error out"=w103:errorcluster, "string"=w122:string, "dup refnum"=w99:refnum<file>)  [unwired: 5 in, 2 out]
        n56 = Bundle("DAQ calibration setup"=w113, "Calibration Channels"=w114) -> (w116:T14)  [unwired: 1 in]
        n57 = local write "Selected Calibration File"(w123) -> ()
        n58 = Unflatten From String(type=w116, binary string=w122) -> (value=w115:T14)  [unwired: 3 in, 2 out]
        n59 = Unbundle(w115) -> ("DAQ calibration setup"=w110:T6, "Calibration Channels"=w107:u16[][])
        "DAQ calibration setup" <- w110
        n60 = Unbundle By Name(w110) -> ("Input Channels"=w109:T15)
        n61 = Array Size(array=w107) -> (size(s)=w111:i32[])
        n62 = Index Array(array=w111, index #1=0 ("index"), index #2=1 ("index")) -> (element #1=w101:i32, element #2=w100:i32)
        n63 = call <vilib>:"Read File+ [I16].vi"("2D number of columns/1D count"=w101, "2D number of rows"=w100, "error in (no error)"=w103, "refnum"=w99) -> ("error out"=w102:errorcluster, "2D data"=w97:i16[][], "dup refnum"=w98:refnum<file>)  [unwired: 2 in, 3 out]
        n64 = To Word Integer(number=w97) -> (16bit integer=w112:i16[][])
        n65 = call <vilib>:"Close File+.vi"("error in (no error)"=w102, "refnum"=w98) -> ()  [unwired: 3 in, 3 out]
        n66 = Transpose 2D Array(2D array=w112) -> (transposed array=w104:i16[][])
        n67 = local write "Cosines fixed"(w104) -> ()
        n68 = for {
          tunnel: w109 -> [w136] mode=indexing
          tunnel: [w135] -> w108 mode=indexing
          n69 = Unbundle By Name(w136) -> ("channel name"=w135:string)
        }
        n70 = stacked-sequence {
          tunnel: w107 -> [w134]
          tunnel: [w134] -> w96
          tunnel: w108 -> [_]
          frame #0 {
          }
        }
        n71 = local write "Calibration Channels"(w96) -> ()
        n72 = Bundle By Name(cluster=w94, "Auto load calibration file"=path "", "Selected Calibration File"=w123, "Cosines fixed"=w104, "Calibration Channels"=w96) -> (w128:T13)
        n73 = property on="cal channel select" class="Ring (strict)"("Strings []"=w108) -> ()  [unwired: 2 in, 2 out]
      }
      frame "SubSample" {
        n74 = case shown="True" "Sub Sample Once" {
          tunnel: w142 -> [w144 w151]
          tunnel: [w144 w145] -> w140
          frame False {
          }
          frame True {
            n75 = Unbundle By Name(w151) -> ("Data File.Data -> 3D Coil"=w147:dbl[][], "Data File.Sample Rate"=w150:i32)
            n76 = for {
              tunnel: w147 -> [w153] mode=indexing
              tunnel: [w152] -> w146 mode=indexing
              n77 = Decimate 1D Array(w153) -> (w152:dbl[])  [unwired: 1 out]
            }
            n78 = Quotient & Remainder(x=w150, y=2) -> (floor(x/y)=w148:i32)  [unwired: 1 out]
            n79 = Bundle By Name(cluster=w151, "Data File.Data -> 3D Coil"=w146, "Data File.Sample Rate"=w148) -> (w145:T13)
          }
        }
        n80 = Unbundle By Name(w140) -> ("Data File"=w139:T8)
        n81 = local write "Data File"(w139) -> ()
      }
      frame "Read 6 Field/Int Data File" {
        w179 = 4 ("count")
        w184 = "/" ("Substring")
        n82 = flat-sequence {
          tunnel: [w191] -> w159
          frame #0 {
            n83 = local read "DC-File"() -> (w192:path)
            n84 = Empty String/Path?(string/path=w192) -> (empty?=w193:bool)
            n85 = case shown="True" w193 {
              tunnel: w192 -> [w194 _]
              tunnel: [w194 w195] -> w191
              frame False {
              }
              frame True {
                n86 = File Dialog(6:"*.raw" ("pattern"), 7:"Select Data File:" ("prompt")) -> (3:w195:path)  [unwired: 5 in, 3 out]
              }
            }
          }
          frame #1 {
            n87 = local write "DC-File"(path "" ("DC-File")) -> ()
          }
        }
        n88 = call <vilib>:"Open_Create_Replace File.vi"("file path"=w159) -> ("refnum"=w182:refnum<file>)  [unwired: 7 in, 3 out]
        n89 = Strip Path(path=w159) -> (stripped path=w158:path, name=w157:string)
        n90 = local read "DAQ data setup"() -> (w177:T6)
        n91 = call <vilib>:"Read File+ (string).vi"("count"=w179, "refnum"=w182) -> ("string"=w180:string, "dup refnum"=w181:refnum<file>)  [unwired: 5 in, 3 out]
        n92 = Strip Path(path=w158) -> (name=w185:string)  [unwired: 1 out]
        n93 = Unflatten From String(type=w179, binary string=w180) -> (value=w178:i32)  [unwired: 3 in, 2 out]
        n94 = Concatenate Strings(w184, w185, w184, w157) -> (w172:string)
        n95 = call <vilib>:"Read File+ (string).vi"("count"=w178, "refnum"=w181) -> ("error out"=w170:errorcluster, "string"=w183:string, "dup refnum"=w171:refnum<file>)  [unwired: 5 in, 2 out]
        n96 = local write "Selected Data File"(w172) -> ()
        n97 = Unflatten From String(type=w177, binary string=w183) -> (value=w176:T6)  [unwired: 3 in, 2 out]
        n98 = Get File Size(file=w171, error in=w170) -> (refnum out=w165:refnum<file>, size (in bytes)=w166:i64, 0:w168:errorcluster)
        n99 = Unbundle By Name(w176) -> ("Sample Rate"=w175:dbl, "Input Channels"=w174:T15)
        n100 = local write "DAQ data setup"(w176) -> ()
        n101 = Array Size(array=w174) -> (size(s)=w169:i32)
        n102 = call <vilib>:"Read File+ [I16].vi"("2D number of columns/1D count"=w169, "2D number of rows"=w166, "error in (no error)"=w168, "refnum"=w165) -> ("error out"=w167:errorcluster, "2D data"=w161:i16[][], "dup refnum"=w164:refnum<file>)  [unwired: 2 in, 3 out]
        n103 = Transpose 2D Array(2D array=w161) -> (transposed array=w160:i16[][])
        n104 = call <vilib>:"Close File+.vi"("error in (no error)"=w167, "refnum"=w164) -> ()  [unwired: 3 in, 3 out]
        n105 = Bundle By Name(cluster=w156, "Experiment data path"=w158, "filename"=w157) -> (w155:T7)
        n106 = To Long Integer(number=w175) -> (32bit integer=w162:i32)
        n107 = To Double Precision Float(number=w160) -> (double precision float=w163:dbl[][])
        n108 = for {
          tunnel: w174 -> [w200] mode=indexing
          tunnel: [w199] -> w173 mode=indexing
          n109 = Unbundle By Name(w200) -> ("channel name"=w199:string)
        }
        n110 = local read "Data File"() -> (w187:T8)
        n111 = Bundle By Name(cluster=w187, "Sample Rate"=w162, "Data -> 3D Coil"=w163) -> (w186:T8)
        n112 = local write "Data File"(w186) -> ()
        n113 = property on="channel select for plot" class="Ring (strict)"("Strings []"=w173) -> ()  [unwired: 2 in, 2 out]
        n114 = property on="channel select" class="Ring (strict)"("Strings []"=w173) -> ()  [unwired: 2 in, 2 out]
        n115 = property on="coil channel select" class="Ring (strict)"("Strings []"=w173) -> ()  [unwired: 2 in, 2 out]
        n116 = Bundle By Name(cluster=w188, "Selected Data File"=w172, "Data File"=w186) -> (w189:T13)
      }
      frame "Sort 6 Field/Int Channels" {
        w217 = dbl[][] []
        n117 = Unbundle By Name(w226) -> ("Calibration Channels"=w208:u16[][], "Cosines fixed"=w209:i16[][], "Data File.Data -> 3D Coil"=w218:dbl[][], "Additional channels"=w219:T5, "Coil Channels"=w213:u16[][], "Channel \nplot"=w215:u16[])
        n118 = Array Size(array=w208) -> (size(s)=w207:i32[])
        n119 = Index Array(array=w207, index #1=0 ("index"), index #2=1 ("index")) -> (element #1=w203:i32, element #2=w204:i32)
        n120 = Multiply(x=w203, y=w204) -> (x*y=w202:i32)
        n121 = Transpose 2D Array(2D array=w213) -> (transposed array=w211:u16[][])
        n122 = Reshape Array(w208, w202) -> (w214:u16[])
        n123 = Reshape Array(w209, w202) -> (w212:i16[])
        n124 = for {
          tunnel: w211 -> [w231] mode=indexing
          tunnel: w214 -> [w230]
          tunnel: w212 -> [w229]
          tunnel: [w228] -> w210 mode=indexing
          n125 = for {
            tunnel: w231 -> [w240] mode=indexing
            tunnel: w230 -> [w236]
            tunnel: w229 -> [w234]
            tunnel: [w232] -> w228 mode=indexing
            n126 = property on="coil channel select" class="Ring (strict)"() -> ("Strings []"=w237:string[])  [unwired: 2 in, 2 out]
            n127 = property on="cal channel select" class="Ring (strict)"() -> ("Strings []"=w239:string[])  [unwired: 2 in, 2 out]
            n128 = Index Array(array=w237, index=w240) -> (element=w238:string)
            n129 = Search 1D Array(1D array=w239, element=w238) -> (index of element=w235:i32)  [unwired: 1 in]
            n130 = Search 1D Array(1D array=w236, element=w235) -> (index of element=w233:i32)  [unwired: 1 in]
            n131 = Index Array(array=w234, index=w233) -> (element=w232:i16)
          }
        }
        n132 = for {
          shift-right: [w280] -> w221
          shift-left: w217 -> [w281]
          tunnel: w218 -> [w275]
          tunnel: w211 -> [w279] mode=indexing
          n133 = Index Array(array=w279, index #1=0 ("index"), index #2=1 ("index"), index #3=2 ("index"), index #4=3 ("index"), index #5=4 ("index"), index #6=5 ("index")) -> (element #1=w274:u16, element #2=w273:u16, element #3=w272:u16, element #4=w264:u16, element #5=w263:u16, element #6=w262:u16)
          n134 = Index Array(array=w275, index (row) #1=w274, index (row) #2=w273, index (row) #3=w272, index (row) #4=w264, index (row) #5=w263, index (row) #6=w262) -> (element #1=w269:dbl[], element #2=w271:dbl[], element #3=w270:dbl[], element #4=w261:dbl[], element #5=w260:dbl[], element #6=w259:dbl[])  [unwired: 6 in]
          n135 = Build Array(w269, w271, w270, w261, w260, w259) -> (w268:dbl[][])
          n136 = Build Array (concatenate)(w281, w268) -> (w280:dbl[][])
        }
        n137 = for {
          tunnel: w219 -> [w258] mode=indexing
          tunnel: w218 -> [w257]
          shift-right: [w250] -> w220
          shift-left: w217 -> [w251]
          n138 = Unbundle By Name(w258) -> ("channel select"=w249:u16, "offset"=w255:dbl, "scale"=w254:dbl)
          n139 = Index Array(array=w257, index (row)=w249) -> (element=w256:dbl[])  [unwired: 1 in]
          n140 = Add(x=w256, y=w255) -> (x+y=w253:dbl[])
          n141 = Multiply(x=w253, y=w254) -> (x*y=w252:dbl[])
          n142 = Build Array (concatenate)(w251, w252) -> (w250:dbl[][])
        }
        n143 = for {
          tunnel: w215 -> [w247] mode=indexing
          tunnel: w218 -> [w248]
          shift-right: [w244] -> w216
          shift-left: w217 -> [w246]
          n144 = Array Subset(array=w248, index (row)=w247, length (row)=1 ("length"), index (col)=0 ("index (row)"), length (col)="plot length") -> (w245:dbl[][])
          n145 = Build Array (concatenate)(w246, w245) -> (w244:dbl[][])
        }
        n146 = local read "Data File"() -> (w223:T8)
        n147 = Bundle By Name(cluster=w223, "Data -> 3D Coil"=w221, "Data -> Additional"=w220, "Data -> Plot"=w216) -> (w222:T8)
        n148 = Bundle By Name(cluster=w226, "Cosines fixed"=w210, "Data File"=w222) -> (w224:T13)
        n149 = local write "Data File"(w222) -> ()
      }
      frame "Calculate 6 Field/Int Rot Matrix" {
        n150 = Unbundle By Name(w312) -> ("Additional channels"=w287:T5, "DAQ data setup.Input Channels"=w286:T15, "Data File.Data -> Additional"=w291:dbl[][], "Data File.Sample Rate"=w294:i32, "Data File.Data -> 3D Coil"=w301:dbl[][], "Data File.Data -> Plot"=w285:dbl[][], "Cosines fixed"=w314:i16[][], "Channel \nplot"=w284:u16[])  [unwired: 1 out]
        n151 = call "JHOC Select Reference.vi"("Channel plot"=w284, "3D Coil"=w285) -> ("References"=w283:i32[])  [unwired: 1 in]
        n152 = for {
          tunnel: w301 -> [w365]
          tunnel: w314 -> [w364]
          tunnel: w283 -> [w360] mode=indexing
          shift-right: [w354] -> w311
          shift-left: dbl[][] [] -> [w356]
          tunnel: ["3D Convention"] -> w310
          i -> [w363]
          w366 = 6 ("x")
          n153 = Multiply(x=w363, y=w366) -> (x*y=w367:i32)
          n154 = Index Array(array=w364, index (row)=w363) -> (element=w361:i16[])  [unwired: 1 in]
          n155 = Array Subset(array=w365, index (row)=w367, length (row)=w366) -> (w362:dbl[][])  [unwired: 2 in]
          n156 = call "3 D Ang Pos for 6 Field-Int.vi"("With Respect To:"=enum16{"Referenced", "UnReferenced"}."Referenced", "LE and RE 2D coils"=FALSE, "Reference index"=w360, "3D Convention"="3D Convention", "Field Gains"=w361, "3D Voltage Data"=w362) -> ("3D Position"=w355:dbl[][])  [unwired: 5 in]
          n157 = Build Array (concatenate)(w356, w355) -> (w354:dbl[][])
        }
        n158 = case shown="False" TRUE {
          tunnel: w311 -> [w337 w348]
          tunnel: w310 -> [w336 w347]
          tunnel: [w335 w341] -> w309
          tunnel: [w334 w341] -> w308
          tunnel: [w333 w341] -> w307
          tunnel: [w332 w338] -> w306
          tunnel: [w331 w346] -> w305
          tunnel: [w330 w341] -> w304
          tunnel: [w329 w342] -> w300
          tunnel: [w328 w342] -> w299
          tunnel: [w327 w342] -> w298
          tunnel: [w326 w345] -> w297
          tunnel: [w325 w344] -> w296
          tunnel: [w324 w342] -> w295
          tunnel: w294 -> [w323 w343]
          frame False {
            n159 = call "Head Co-ordinates 2.vi"("3D Convention"=w336, "3D Type and Co-ordinate System"=T11."Position in Space", "Array"=w337) -> ("Channel List"=w329:string[], "3D Output"=w335:dbl[][])  [unwired: 3 in]
            n160 = call "Head Co-ordinates 2.vi"("3D Convention"=w336, "3D Type and Co-ordinate System"=T11."Position in Head", "Array"=w337) -> ("Channel List"=w326:string[], "3D Output"=w332:dbl[][])  [unwired: 3 in]
            n161 = call "Head Co-ordinates 2.vi"("3D Convention"=w336, "3D Type and Co-ordinate System"=T11."Velocity in Space", "Sample Rate"=w323, "Array"=w335) -> ("Channel List"=w328:string[], "3D Output"=w334:dbl[][])  [unwired: 2 in]
            n162 = call "Head Co-ordinates 2.vi"("3D Convention"=w336, "3D Type and Co-ordinate System"=T11."Velocity in Head", "Sample Rate"=w323, "Array"=w332) -> ("Channel List"=w325:string[], "3D Output"=w331:dbl[][])  [unwired: 2 in]
            n163 = call "Head Co-ordinates 2.vi"("3D Type and Co-ordinate System"=T11."Acceleration in Space", "Sample Rate"=w323, "Array"=w334) -> ("Channel List"=w327:string[], "3D Output"=w333:dbl[][])  [unwired: 3 in]
            n164 = call "Head Co-ordinates 2.vi"("3D Type and Co-ordinate System"=T11."Acceleration in Head", "Sample Rate"=w323, "Array"=w331) -> ("Channel List"=w324:string[], "3D Output"=w330:dbl[][])  [unwired: 3 in]
          }
          frame True {
            w341 = dbl[][] [] ("3D Output")
            w342 = string[] [] ("Channel List")
            n165 = call "Head Co-ordinates 2.vi"("3D Convention"=w347, "3D Type and Co-ordinate System"=T11."Position in Head", "Array"=w348) -> ("Channel List"=w345:string[], "3D Output"=w338:dbl[][])  [unwired: 3 in]
            n166 = call "Head Co-ordinates 2.vi"("3D Convention"=w347, "3D Type and Co-ordinate System"=T11."Velocity in Head", "Sample Rate"=w343, "Array"=w338) -> ("Channel List"=w344:string[], "3D Output"=w346:dbl[][])  [unwired: 2 in]
          }
        }
        n167 = for {
          tunnel: w287 -> [w353] mode=indexing
          tunnel: w286 -> [w352]
          tunnel: [w349] -> w292 mode=indexing
          n168 = Unbundle By Name(w353) -> ("channel select"=w351:u16)
          n169 = Index Array(array=w352, index=w351) -> (element=w350:T16)
          n170 = Unbundle By Name(w350) -> ("channel name"=w349:string)
        }
        n171 = Build Array (concatenate)(w300, w299, w298, w297, w296, w295, w292, string[] [" "] ("Input Array")) -> (w289:string[])
        n172 = property on="Ring" class="Ring (strict)"("Strings []"=w289) -> ()  [unwired: 2 in, 2 out]
        n173 = Build Array (concatenate)(w309, w308, w307, w306, w305, w304, w291) -> (w303:dbl[][])
        n174 = Bundle By Name(cluster=w312, "All Data.Data Channels"=w303, "DAQ data setup.Sample Rate"=w294, "All Data.Channel List"=w289) -> (w302:T13)
        n175 = Unbundle By Name(w302) -> ("All Data"=w288:T9)
        n176 = local write "All Data"(w288) -> ()
      }
      frame "Export Channels" {
        n177 = Unbundle By Name(w378) -> ("DAQ data setup.Sample Rate"=w379:dbl, "All Data.Data Channels"=w377:dbl[][], "All Data.Channel List"=w374:string[])
        n178 = for {
          tunnel: w377 -> [w386]
          tunnel: "Export Channel List" -> [w383] mode=indexing
          tunnel: [w385] -> w375 mode=indexing
          tunnel: w374 -> [w384]
          tunnel: [w382] -> w369 mode=indexing
          n179 = Index Array(array=w384, index=w383) -> (element=w382:string)
          n180 = Index Array(array=w386, index (row)=w383) -> (element=w385:dbl[])  [unwired: 1 in]
        }
        n181 = Bundle By Name(cluster=w373, "Data File.Sample Rate"=w379, "Data File.Data Channels"=w375, "Data File.Channel List"=w369, "Parameter Time Series"="Parameter Time Series", "Parameter Impuls Series"="Parameter Impuls Series", "Experiment Parameters"=T12 {"Freq"=0.0, "Vel"=0, "Acc"=0, "Stimulus"="Head Impulse"}) -> (w372:T7)
        n182 = property on="List 1" class="Ring (strict)"("Strings []"=w369) -> ()  [unwired: 2 in, 2 out]
        n183 = property on="Channel" class="Ring (strict)"("Strings []"=w369) -> ()  [unwired: 2 in, 2 out]
      }
      frame "Stop" {
      }
      frame "Quit", Default {
      }
    }
  }
  "Statemachine Data IN 2" <- w1
